vi "Write stop if true.vi"(5 "stop if true":bool, 9 "ForLoop in":refnum<class "WhileLoop.lvclass">) -> (3 "ForLoop out":refnum<class "WhileLoop.lvclass">)   [LabVIEW 2014, in "Raspberry Pi Compatible Compiler for LabVIEW.lvlib" / "WhileLoop.lvclass"]
uses:
  WhileLoop.lvclass
  WhileLoop.lvclass/WhileLoop.ctl
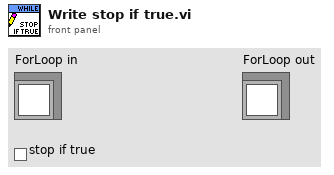
[diagram p1: front panel]
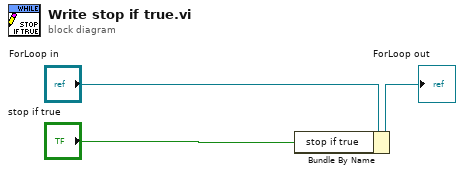
[diagram p0: block diagram]
diagram:
  n1 = Bundle By Name(cluster="ForLoop in", "stop if true"="stop if true") -> (→"ForLoop out":refnum<class "WhileLoop.lvclass">)
